vi "Async Engine.vi"(10 "Parameters":variant, 11 "Process":refnum<class "Process.lvclass">) -> ()   [LabVIEW 2017, in "NI 272x Resistive Simulation Custom Device Engine.lvlib"]
uses:
  NI 272x Resistive Simulation Custom Device Engine.lvlib
  <vilib>/NI/NIVS Inline Async API/_VS Inline Async API/Process/Process.lvclass
  Controls/Compiled Engine Data.ctl
  Controls/Compiled HW Channel.ctl
  Controls/Channel Mode.ctl
  <instrlib>/ni272xReferenceVIs/ni272xReferenceVIs.llb/ni272x Callendar-Van Dusen RTD Parameters.ctl
  Controls/Compiled Connect Channel.ctl
  <vilib>/NI/NIVS Inline Async API/_VS Inline Async API/Process/Process.lvclass/Process.ctl
  <vilib>/Platform/TimedLoop/XDataNode/timing_clust.ctl
  <vilib>/Platform/TimedLoop/XDataNode/nitl_modes.ctl
  <vilib>/Platform/TimedLoop/XDataNode/wakeup.ctl
  <vilib>/NI/NIVS Inline Async API/_Data Access Engine/Access Type Classes/Read/Read.lvclass/Read.ctl
  <vilib>/NI/NIVS Inline Async API/_Data Access Engine/Access Type Classes/Write/Write.lvclass/Write.ctl
  <vilib>/NI/NIVS Inline Async API/_Data Access Engine/Data Access Engine/Methods/Read.Data.vi
  <vilib>/NI/NIVS Inline Async API/_Data Access Engine/Data Access Engine/Methods/Write.Data.vi
  <vilib>/NI/NIVS Inline Async API/_VS Inline Async API/Process/Data Member Access/Read Data Access.vi
  <vilib>/NI/NIVS Inline Async API/_VS Inline Async API/Error Handling Process/SubVIs/Error.ConvertArray.vi
  <vilib>/NI/NIVS Inline Async API/_Data Access Engine/Access Type Classes/Read/Read.ProcessData.vi
  <vilib>/NI/NIVS Inline Async API/_Data Access Engine/Access Type Classes/Write/Write.ProcessData.vi
  <vilib>/NI/NIVS Inline Async API/_Data Access Engine/Data Access Engine/Methods/Write.Lookup.vi
  <vilib>/NI/NIVS Inline Async API/_Data Access Engine/Data Access Engine/Methods/Read.Lookup.vi
  <vilib>/NI/NIVS Inline Async API/_Data Access Engine/Data Access Engine/Data Access Engine.lvclass
  <vilib>/Platform/TimedLoop/XDataNode/XDataNode.xnode
  <vilib>/Platform/TimedLoop/XDataNode/XDNodeRunTimeDep.lvlib
  NI 272x Resistive Simulation Custom Device Shared.lvlib
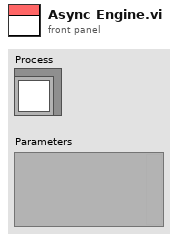
[diagram p1: front panel]
types:
  T1 = typedef "NI 272x Resistive Simulation Custom Device Shared.lvlib/Compiled Engine Data.ctl" = cluster{"HW Chns":T2[], "Con Chns":T5[], "DevName":string, "TL dt":i64}
  T2 = typedef "NI 272x Resistive Simulation Custom Device Shared.lvlib/Compiled HW Channel.ctl" = cluster{"Mode":T3, "RTD":T4, "Last Des Val":dbl, "HW CH":string}
  T3 = typedef "NI 272x Resistive Simulation Custom Device Shared.lvlib/Channel Mode.ctl" = enum16{"Resistance", "RTD Temperature"}
  T4 = typedef "ni272x Callendar-Van Dusen RTD Parameters.ctl" = cluster{"A":dbl, "B":dbl, "C":dbl, "R0":dbl}
  T5 = typedef "NI 272x Resistive Simulation Custom Device Shared.lvlib/Compiled Connect Channel.ctl" = cluster{"HW CH":string, "Is Con":bool, "HW CH+1":string}
  T6 = typedef "Data Access Engine.lvlib/Data Access Engine.lvclass/Write.DVR.ctl" = refnum<data-value>
  T7 = typedef "Data Access Engine.lvlib/Data Access Engine.lvclass/Read.DVR.ctl" = refnum<data-value>
  T8 = typedef "XDNodeRunTimeDep.lvlib/timing_clust.ctl" = cluster{"Expected End [f-1]":u64, "Actual End [f-1]":u64, "Finished Late? [f-1]":bool, "Expected End [i-1]":u64, "Actual End [i-1]":u64, "Finished Late? [i-1]":bool, "Expected Start [i]":u64, "Actual Start [i]":u64, "Expected Start [f]":u64, "Actual Start [f]":u64, "Source Name":string, "Structure Name":string, "Period":i64, "Deadline":i64, "Offset":i64, "Start":i64, "Priority":i32, "Timeout":i32, "Mode":T9, "Wakeup Reason":T10, "Error":errorcluster, "Source Type":string, "Secondary Source Type":string, "Global End Time":u64, "Global Start Time":u64, "Frame Duration":u64, "Iteration Duration":u64, "Assigned CPU":i32, "I/O Scan Engine Mode":u32}
  T9 = typedef "XDNodeRunTimeDep.lvlib/nitl_modes.ctl" = enum32{"No Change", "Process missed periods, maintain original phase", "Discard missed periods, maintain original phase", "Process missed periods, ignore original phase", "Discard missed periods, ignore original phase"}
  T10 = typedef "XDNodeRunTimeDep.lvlib/wakeup.ctl" = enum32{"Normal", "Aborted", "Asynchronous wakeup", "Timing source error", "Timed loop error", "Timeout"}
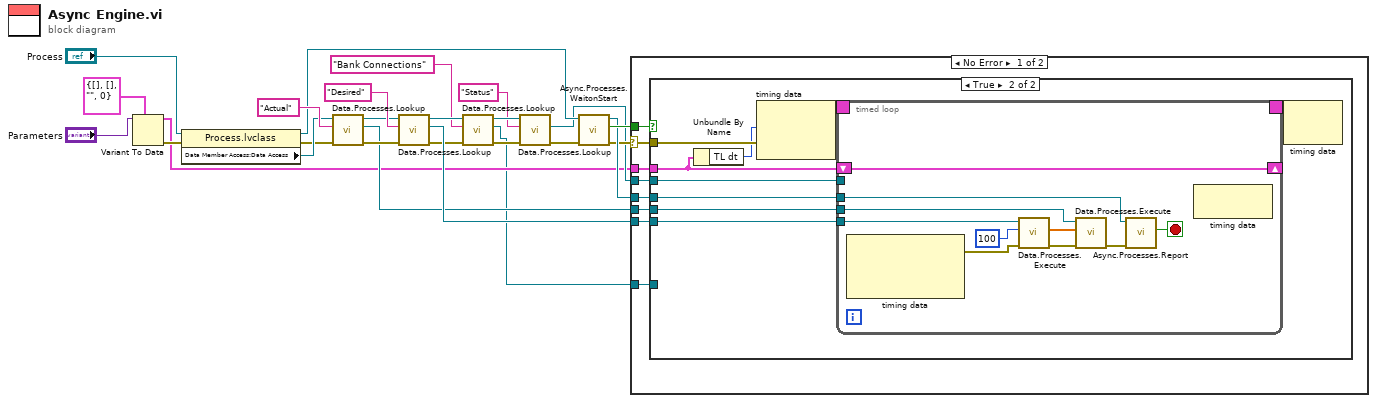
[diagram p0: block diagram]
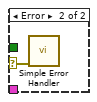
[diagram p3: hidden frame]
diagram:
  n1 = Variant To Data(type=T1 {"HW Chns"=[], "Con Chns"=[], "DevName"="", "TL dt"=0} ("Compiled Engine Data"), Variant="Parameters") -> (data=w2:T1, error out=w3:errorcluster)  [unwired: 1 in]
  n2 = property class="Process.lvclass"(reference="Process", error in=w3) -> (reference out=w17:refnum<class "Process.lvclass">, error out=w15:errorcluster, "Data Member Access:Data Access"=w16:refnum<class "Data Access Engine.lvclass">)
  n3 = call-poly <vilib>:"Data.Processes.Lookup.vi"("error in (no error)"=w15, "Name"="Actual", "Data Access API in"=w16) -> ("error out"=w20:errorcluster, "Ref"=w19:T6, "Data Access API out"=w18:refnum<class "Data Access Engine.lvclass">)  [unwired: 5 in, 1 out]
  n4 = call-poly <vilib>:"Data.Processes.Lookup.vi"("error in (no error)"=w20, "Name"="Desired", "Data Access API in"=w18) -> ("error out"=w9:errorcluster, "Ref"=w22:T7, "Data Access API out"=w13:refnum<class "Data Access Engine.lvclass">)  [unwired: 5 in, 1 out]
  n5 = call-poly <vilib>:"Data.Processes.Lookup.vi"("error in (no error)"=w9, "Name"="Bank Connections", "Data Access API in"=w13) -> ("error out"=w8:errorcluster, "Ref"=w1:T7, "Data Access API out"=w12:refnum<class "Data Access Engine.lvclass">)  [unwired: 5 in, 1 out]
  n6 = call-poly <vilib>:"Data.Processes.Lookup.vi"("error in (no error)"=w8, "Name"="Status", "Data Access API in"=w12) -> ("error out"=w7:errorcluster, "Ref"=w6:T6)  [unwired: 5 in, 2 out]
  n7 = call <vilib>:"Async.Processes.WaitonStart.vi"("error in (no error)"=w7, "Process"=w17) -> ("error out"=w24:errorcluster, "Execute"=w26:bool, "Process out"=w25:refnum<class "Process.lvclass">)  [unwired: 7 in]
  n8 = case shown="No Error" w24 {
    selector: w24 -> [w30 w62]
    tunnel: w26 -> [w34 _]
    tunnel: w25 -> [w33 _]
    tunnel: w19 -> [w32 _]
    tunnel: w22 -> [w31 _]
    tunnel: w2 -> [w29 _]
    tunnel: w6 -> [w28 _]
    tunnel: w1 -> [w27 _]
    frame No Error {
      n9 = case shown="True" w34 {
        tunnel: w30 -> [_ w38]
        tunnel: w33 -> [_ w41]
        tunnel: w31 -> [_ w43]
        tunnel: w32 -> [_ w42]
        tunnel: w29 -> [_ w37]
        tunnel: w28 -> [_ w35]
        tunnel: w27 -> [_ _]
        frame False {
        }
        frame True {
          n10 = Unbundle By Name(w37) -> ("TL dt"=w36:i64)
          n11 = node-c288(w36, w38) -> (w40:T8)
          n12 = timed-loop {
            tunnel: w41 -> [w53]
            tunnel: w43 -> [w51]
            tunnel: w42 -> [w50]
            timing: w40 -> [_]
            timing-out: [_] -> w39
            shift-right: [w44] -> _
            shift-left: w37 -> [w44]
            tunnel: w35 -> [_]
            stop <- w52 stop-if-true
            n13 = node-c288() -> (w45:errorcluster)  [unwired: 1 in, 2 out]
            n14 = call-poly <vilib>:"Data.Processes.Execute.vi"("error in (no error)"=w45, "timeout ms"=100, "Ref"=w51) -> ("error out"=w46:errorcluster, "Values"=w47:dbl[])  [unwired: 6 in, 1 out]
            n15 = call-poly <vilib>:"Data.Processes.Execute.vi"("error in (no error)"=w46, "Values"=w47, "Ref"=w50) -> ("error out"=w48:errorcluster)  [unwired: 8 in]
            n16 = call <vilib>:"Async.Processes.Report.vi"("Error"=w48, "Process in"=w53) -> ("Stop"=w52:bool)  [unwired: 8 in, 1 out]
            n17 = node-c288() -> ()  [unwired: 1 in, 1 out]
          }
          n18 = node-c288(w39) -> ()  [unwired: 1 out]
        }
      }
    }
    frame Error {
      n19 = call <vilib>:"Simple Error Handler.vi"("error in (no error)"=w62) -> ()  [unwired: 4 in, 5 out]
    }
  }
